vi "Get Ctrl Ref.vi"(0 "VI Reference In":refnum<vi>, 5 "Control Path":string, 11 "Error In":errorcluster) -> (4 "VI Reference Out":refnum<vi>, 6 "Ctl Refnum":refnum<vi>, 15 "Error Out":errorcluster)   [LabVIEW 2019, in "SLL JSON to Cluster.lvlib"]
doc: "This VI fetches the ctrl refernce of the given ctrl label from for the input VI reference."
uses:
  SLL JSON to Cluster.lvlib
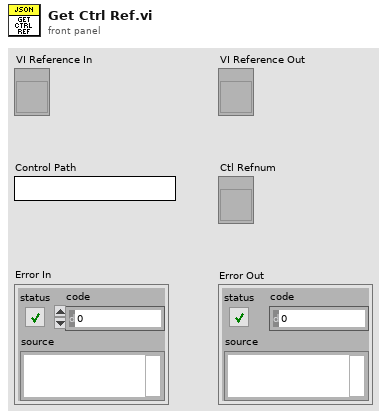
[diagram p1: front panel]
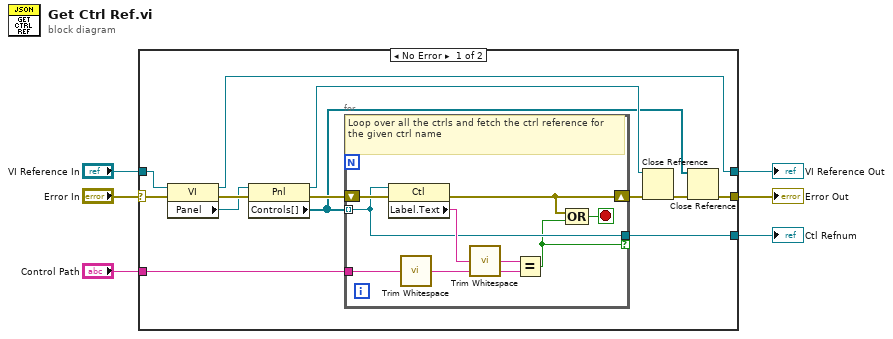
[diagram p0: block diagram]
diagram:
  n1 = case shown="No Error" "Error In" {
    selector: "Error In" -> [w17 w30]
    tunnel: "Control Path" -> [w14 _]
    tunnel: [w8 w30] -> w5
    tunnel: "VI Reference In" -> [w16 w29]
    tunnel: [w7 w29] -> w2
    tunnel: [w13 _] -> w1
    frame No Error {
      n2 = property class="VI"(reference=w16, error in=w17) -> (reference out=w7:refnum<vi>, error out=w19:errorcluster, "Panel"=w18:refnum<vi>)
      n3 = property class="Pnl"(reference=w18, error in=w19) -> (reference out=w11:refnum<vi>, error out=w15:errorcluster, "Controls[]"=w9:refnum<vi>[])
      n4 = for {
        shift-right: [w24] -> w12
        shift-left: w15 -> [w28]
        tunnel: w9 -> [w25] mode=indexing
        tunnel: w14 -> [w27]
        tunnel: [w25] -> w13 if=w22
        stop <- w23 stop-if-true
        # "Loop over all the ctrls and fetch the ctrl reference for the given ctrl name"
        n5 = property class="Ctl"(reference=w25, error in=w28) -> (error out=w24:errorcluster, "Label.Text"=w26:string)  [unwired: 1 out]
        n6 = call <vilib>:"Trim Whitespace.vi"("string"=w27) -> ("trimmed string"=w20:string)  [unwired: 1 in]
        n7 = call <vilib>:"Trim Whitespace.vi"("string"=w26) -> ("trimmed string"=w21:string)  [unwired: 1 in]
        n8 = Equal?(x=w21, y=w20) -> (x = y?=w22:bool)
        n9 = Compound Arithmetic op=OR(w24, w22) -> (w23:bool)
      }
      n10 = Close Reference(reference=w11, error in (no error)=w12) -> (error out=w10:errorcluster)
      n11 = Close Reference(reference=w9, error in (no error)=w10) -> (error out=w8:errorcluster)
    }
    frame Error {
    }
  }
  "Ctl Refnum" <- w1
  "Error Out" <- w5
  "VI Reference Out" <- w2
